vi "FindErrorsUsingText.vi"(8 "ErrorIn":errorcluster caption="Error In(no Error)", 9 "SearchTexts":string[](array[string]), 11 "ReferenceIn":refnum<class "ErrorDefinitionSQLite.lvclass"> caption="Reference In") -> (0 "ErrorOut":errorcluster caption="Error Out", 1 "Errors":T1, 3 "ReferenceOut":refnum<class "ErrorDefinitionSQLite.lvclass"> caption="Reference Out")   [LabVIEW 2018, in "ErrorDefinitionSQLite.lvclass"]
uses:
  ErrorDefinitionSQLite.lvclass
  ErrorContent.ctl
  <vilib>/drjdpowell/SQLite Library/SQL Connection/Open (path).vi
  <vilib>/drjdpowell/SQLite Library/SQL Connection/Open (string).vi
  <vilib>/AdvancedString/Path To Command Line String.vi
  <vilib>/drjdpowell/SQLite Library/SQL Connection/Execute SQL.vi
  <vilib>/drjdpowell/SQLite Library/SQL Connection/Connection.lvclass
  <vilib>/drjdpowell/SQLite Library/SQLite.lvlib
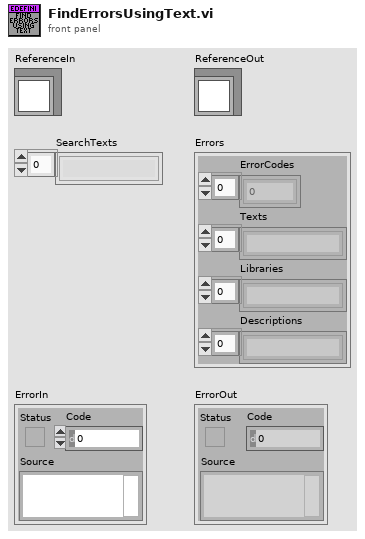
[diagram p1: front panel]
types:
  T1 = typedef "ErrorDefinitionSQLite.lvclass/ErrorContent.ctl" = cluster{"ErrorCodes":i32[], "Texts":string[], "Libraries":string[], "Descriptions":string[]}
  T2 = enum16{"New or existing", "Existing", "Read only"}
  T3 = typedef "ErrorDefinitionSQLite.lvclass/ObjectAttributes.ctl" = cluster{"Path":path}
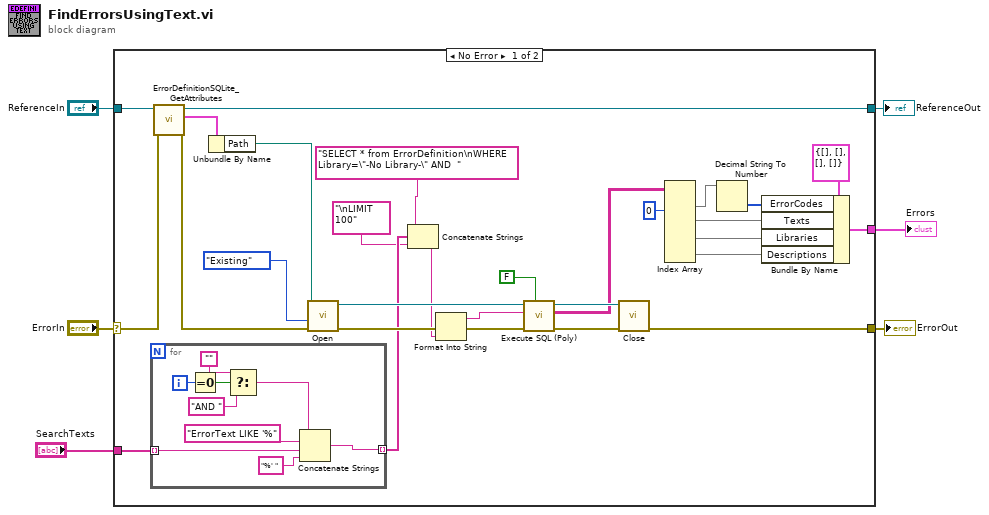
[diagram p0: block diagram]
diagram:
  n1 = case shown="No Error" "ErrorIn" {
    selector: "ErrorIn" -> [w35 w46]
    tunnel: [w21 w46] -> w5
    tunnel: [w33 w45] -> w3
    tunnel: "ReferenceIn" -> [w34 w45]
    tunnel: "SearchTexts" -> [w11 _]
    tunnel: [w12 _] -> w2
    frame No Error {
      n2 = for {
        tunnel: w11 -> [w44] mode=indexing
        tunnel: [w41] -> w9 mode=indexing
        i -> [w40]
        n3 = Equal To 0?(x=w40) -> (x = 0?=w39:bool)
        n4 = Select(t="", s=w39, f="AND " ("string")) -> (s? t:f=w36:string)
        n5 = Concatenate Strings(w36, "ErrorText LIKE '%" ("string"), w44, "%' " ("string")) -> (w41:string)
      }
      n6 = call "ErrorDefinitionSQLite_GetAttributes.vi"("ErrorIn"=w35, "Reference in"=w34) -> ("ErrorOut"=w29:errorcluster, "Data"=w31:T3, "Reference out"=w33:refnum<class "ErrorDefinitionSQLite.lvclass">)  [unwired: 6 in, 1 out]
      n7 = Unbundle By Name(w31) -> ("Path"=w30:path)
      n8 = call-poly <vilib>:"Open.vi"("error in (no error)"=w29, "File Option"=T2."Existing", "db file"=w30) -> ("error out"=w25:errorcluster, "SQLite Connection"=w27:refnum<class "Connection.lvclass">)  [unwired: 7 in]
      n9 = Concatenate Strings("SELECT * from ErrorDefinition\nWHERE Library=\"-No Library-\" AND  " ("SQL"), w9, "\nLIMIT 100" ("SQL")) -> (w8:string)
      n10 = Format Into String(error in=w25, w8) -> (resulting string=w26:string, error out=w24:errorcluster)  [unwired: 2 in]
      n11 = call-poly <vilib>:"Execute SQL (Poly).vi"("Use SAVEPOINT"=FALSE, "error in (no error)"=w24, "SQL"=w26, "SQLite Connection in"=w27) -> ("error out"=w22:errorcluster, "Result Set"=w20:string[][], "SQLite Connection"=w23:refnum<class "Connection.lvclass">)  [unwired: 4 in, 1 out]
      n12 = call-dynamic "Close.vi"("error in (no error)"=w22, "SQLite Connection in"=w23) -> ("error out"=w21:errorcluster)  [unwired: 9 in]
      n13 = Index Array(array=w20, index (col) #1=0 ("disabled index (col)")) -> (element #1=w14:string[], element #2=w15:string[], element #3=w16:string[], element #4=w17:string[])  [unwired: 7 in]
      n14 = Decimal String To Number(string=w14) -> (number=w13:i32[])  [unwired: 2 in, 1 out]
      n15 = Bundle By Name(cluster=T1 {"ErrorCodes"=[], "Texts"=[], "Libraries"=[], "Descriptions"=[]} ("Errors"), "ErrorCodes"=w13, "Texts"=w15, "Libraries"=w16, "Descriptions"=w17) -> (w12:T1)
    }
    frame Error {
    }
  }
  "ErrorOut" <- w5
  "ReferenceOut" <- w3
  "Errors" <- w2
